vi "Track Voltage and Current.vi"() -> ()   [LabVIEW 2014]
panel:
  out "Hardware Fault":bool
  out "Temperature Fault":bool
  out "Battery Voltage Fault":bool
  out "Current Faults":bool[](array[boolean])
  out "Power (W)":dbl
  out "Energy (J)":dbl
  out "voltage (V)":dbl
  out "all currents (A)":dbl[](array[numeric])
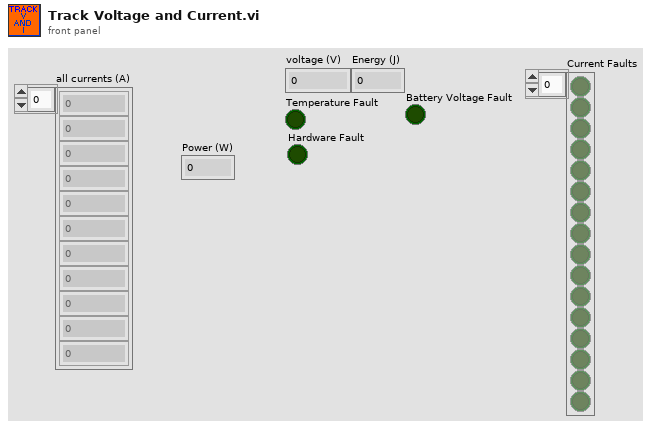
[diagram p1: front panel]
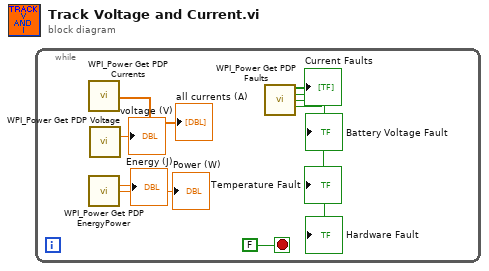
[diagram p0: block diagram]
diagram:
  n1 = while {
    stop <- FALSE stop-if-true
    n2 = call <vilib>:"WPI_Power Get PDP Currents.vi"() -> ("all currents (A)"=→"all currents (A)":dbl[])  [unwired: 13 in, 2 out]
    n3 = call <vilib>:"WPI_Power Get PDP EnergyPower.vi"() -> ("Energy (J)"=→"Energy (J)":dbl, "Power (W)"=→"Power (W)":dbl)  [unwired: 13 in, 1 out]
    n4 = call <vilib>:"WPI_Power Get PDP Voltage.vi"() -> ("voltage (V)"=→"voltage (V)":dbl)  [unwired: 14 in, 1 out]
    n5 = call <vilib>:"WPI_Power Get PDP Faults.vi"() -> ("Current Faults"=→"Current Faults":bool[], "Battery Voltage Fault"=→"Battery Voltage Fault":bool, "Temperature Fault"=→"Temperature Fault":bool, "Hardware Fault"=→"Hardware Fault":bool)  [unwired: 11 in, 1 out]
  }
